vi "GUID string to int.vi"(11 "uuid":string) -> (3 "GUID":T1 {"Lo" format="%.0x"; "Hi" format="%.0x"})   [LabVIEW 2013, in "NISE_CEF_serializable configuration.lvclass"]
uses:
  NISE_CEF_serializable configuration.lvclass
  Numeric GUID.ctl
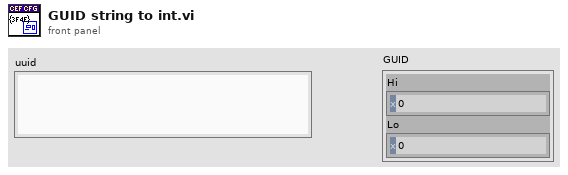
[diagram p1: front panel]
types:
  T1 = typedef "NISE_CEF_serializable configuration.lvclass/Numeric GUID.ctl" = cluster{"Hi":u64, "Lo":u64}
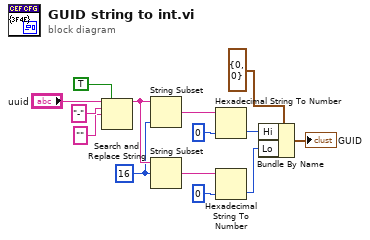
[diagram p0: block diagram]
diagram:
  w1 = 16 ("length (rest)")
  n1 = Search and Replace String(replace all?=TRUE ("replace all? (F)"), input string="uuid", search string="-" ("new element/subarray"), replace string="" ("replace string (\"\")")) -> (result string=w4:string)  [unwired: 4 in, 3 out]
  n2 = String Subset(string=w4, length (rest)=w1) -> (substring=w3:string)  [unwired: 1 in]
  n3 = String Subset(string=w4, offset (0)=w1) -> (substring=w2:string)  [unwired: 1 in]
  n4 = Hexadecimal String To Number(string=w3, default (0uL)=u64 0 ("default (0 U32)")) -> (number=w11:u64)  [unwired: 1 in, 1 out]
  n5 = Hexadecimal String To Number(string=w2, default (0uL)=u64 0 ("default (0 U32)")) -> (number=w10:u64)  [unwired: 1 in, 1 out]
  n6 = Bundle By Name(cluster=T1 {"Hi"=0, "Lo"=0} ("GUID"), "Hi"=w11, "Lo"=w10) -> (→"GUID":T1)
